vi "XVA-DSE7-dist.vi"(8 "err in":errorcluster, 10 "X-VA (e)":T2, 11 "p_LW":T1) -> (0 "err out":errorcluster, 2 "VA (s)":T2, 3 "p_LW (s)":T1)   [LabVIEW 2010, in "lv_04.lvlib"]
uses:
  lv_04.lvlib
  commandes/cX.ctl
  commandes/cSTA_varid.ctl
  commandes/c_TDMS_ch_variable.ctl
  commandes/c_TDMS_ch_donnees.ctl
  commandes/c0-var-n.ctl
  commandes/cSTA_num_do_cr.ctl
  commandes/c02-do-num.ctl
  commandes/c04-stat-num.ctl
  commandes/cSTA_txt_do_cr.ctl
  commandes/c02-do-txt.ctl
  commandes/c04-stat-txt.ctl
  commandes/cSTA_dist.ctl
  commandes/c03-dist-S.ctl
  commandes/c0-dist-xy.ctl
  commandes/c03-dist-T.ctl
  commandes/c03-dist-SPC.ctl
  lv_02/p_5E7_LW.ctl
  lv_02/7-t-dist.vi
  lv_02/lv_02.lvlib
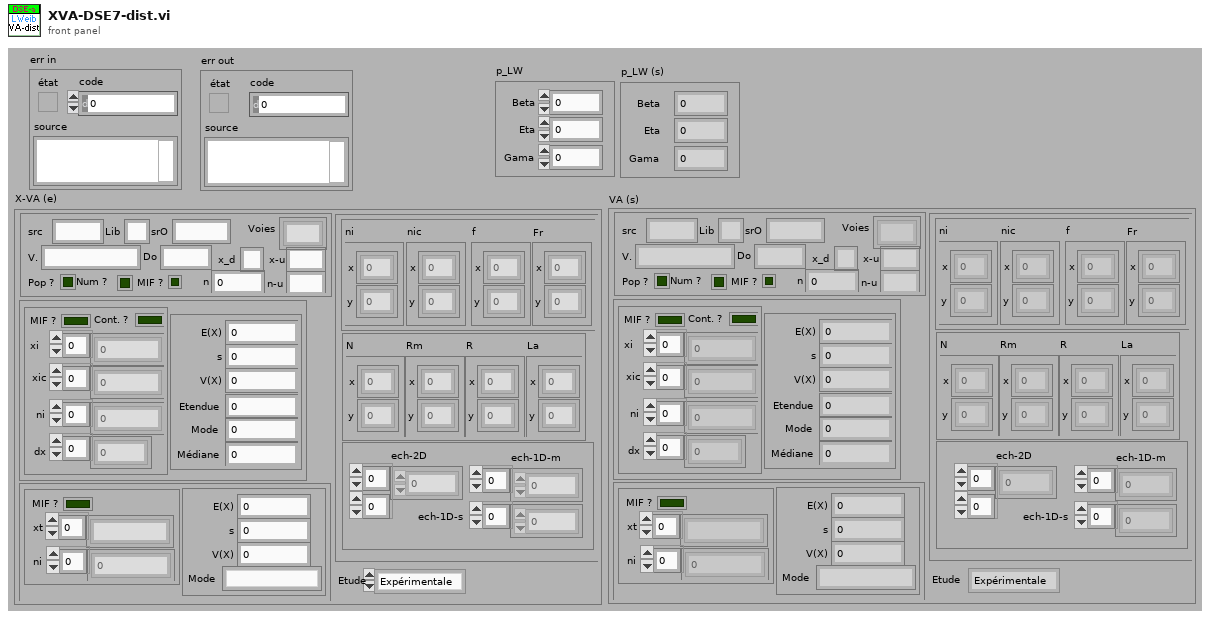
[diagram p1: front panel]
types:
  T1 = typedef "lv_02.lvlib/p_5E7_LW.ctl" = cluster{"Beta":dbl, "Eta":dbl, "Gama":dbl}
  T2 = typedef "lv_04.lvlib/cX.ctl" = cluster{"src":T3, "num":T7, "txt":T10, "dist":T13, "Etude":enum16{"Expérimentale", "Modèle"}}
  T3 = typedef "lv_04.lvlib/cSTA_varid.ctl" = cluster{"src":string, "Lib":string, "srO":string, "V.":T4, "Voies":string[], "Do":T5, "n":T6, "Num ?":bool, "Pop ?":bool, "x_d":string, "x-u":string, "n-u":string, "MIF ?":bool}
  T4 = typedef "lv_04.lvlib/c_TDMS_ch_variable.ctl" = string
  T5 = typedef "lv_04.lvlib/c_TDMS_ch_donnees.ctl" = string
  T6 = typedef "lv_04.lvlib/c0-var-n.ctl" = i32
  T7 = typedef "lv_04.lvlib/cSTA_num_do_cr.ctl" = cluster{"do":T8, "sta":T9}
  T8 = typedef "lv_04.lvlib/c02-do-num.ctl" = cluster{"MIF ?":bool, "Cont. ?":bool, "xi":dbl[], "xic":dbl[], "ni":u32[], "dx":dbl[]}
  T9 = typedef "lv_04.lvlib/c04-stat-num.ctl" = cluster{"E(X)":dbl, "s":dbl, "V(X) ":dbl, "Etendue":dbl, "Mode":dbl, "Médiane":dbl}
  T10 = typedef "lv_04.lvlib/cSTA_txt_do_cr.ctl" = cluster{"do":T11, "sta":T12}
  T11 = typedef "lv_04.lvlib/c02-do-txt.ctl" = cluster{"xt":string[], "ni":dbl[], "MIF ?":bool}
  T12 = typedef "lv_04.lvlib/c04-stat-txt.ctl" = cluster{"E(X)":dbl, "s":dbl, "V(X) ":dbl, "Mode":string}
  T13 = typedef "lv_04.lvlib/cSTA_dist.ctl" = cluster{"S":T14, "T":T16, "spc":T17}
  T14 = typedef "lv_04.lvlib/c03-dist-S.ctl" = cluster{"nic":T15, "f":T15, "Fr":T15, "ni":T15}
  T15 = typedef "lv_04.lvlib/c0-dist-xy.ctl" = cluster{"x":dbl[], "y":dbl[]}
  T16 = typedef "lv_04.lvlib/c03-dist-T.ctl" = cluster{"N":T15, "Rm":T15, "R":T15, "La":T15}
  T17 = typedef "lv_04.lvlib/c03-dist-SPC.ctl" = cluster{"ech-2D":dbl[][], "ech-1D-m":dbl[], "ech-1D-s":dbl[]}
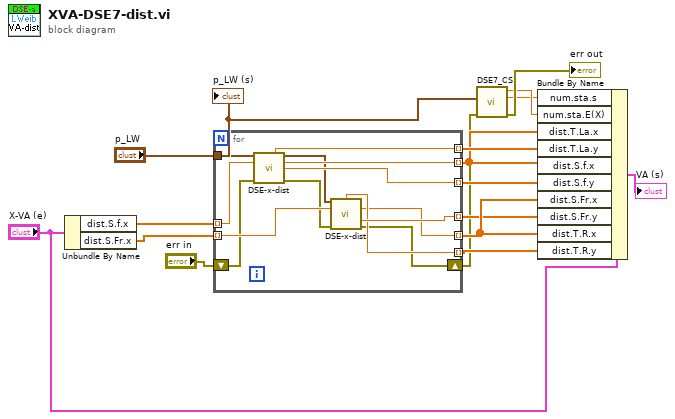
[diagram p0: block diagram]
diagram:
  n1 = Unbundle By Name("X-VA (e)") -> ("dist.S.f.x"=w14:dbl[], "dist.S.Fr.x"=w13:dbl[])
  n2 = for {
    tunnel: [w29] -> w12 mode=indexing
    tunnel: [w28] -> w15 mode=indexing
    tunnel: [w27] -> w11 mode=indexing
    tunnel: [w22] -> w8 mode=indexing
    shift-right: [w19] -> w4
    shift-left: "err in" -> [w17]
    tunnel: "p_LW" -> [w26]
    tunnel: w14 -> [w25] mode=indexing
    tunnel: w13 -> [w23] mode=indexing
    tunnel: [w21] -> w10 mode=indexing
    tunnel: [w20] -> w9 mode=indexing
    n3 = call-poly "DSE-x-dist.vi"("p_LW"=w26, "t"=w25, "error in"=w17) -> ("La (t)"=w28:dbl, "p_LW"=w24:T1, "t"=w29:dbl, "f (t)"=w27:dbl, "error out"=w18:errorcluster)  [unwired: 6 in, 2 out]
    n4 = call-poly "DSE-x-dist.vi"("p_LW"=w24, "t"=w23, "error in"=w18) -> ("R(t)"=w21:dbl, "t"=w20:dbl, "F (t)"=w22:dbl, "error out"=w19:errorcluster)  [unwired: 6 in, 3 out]
  }
  n5 = call "DSE7_CS.vi"("error in (no error)"=w4, "Weibull (paramètres)"="p_LW") -> ("error out"=→"err out":errorcluster, "sigma"=w1:dbl, "MTTF"=w2:dbl)  [unwired: 7 in]
  n6 = Bundle By Name(cluster="X-VA (e)", "num.sta.s"=w1, "num.sta.E(X)"=w2, "dist.T.La.x"=w12, "dist.T.La.y"=w15, "dist.S.f.x"=w12, "dist.S.f.y"=w11, "dist.S.Fr.x"=w9, "dist.S.Fr.y"=w8, "dist.T.R.x"=w9, "dist.T.R.y"=w10) -> (→"VA (s)":T2)
  "p_LW (s)" <- "p_LW"
